vi "unweightedStats.vi"(7 "U":dbl[](array[numeric]), 9 "Data Shift Input":dbl[](array[numeric])) -> (0 "Skew":dbl, 1 "Kurt":dbl, 2 "u'/U":dbl, 3 "u^4":dbl, 4 "U":dbl, 5 "u^3":dbl, 6 "u^2":dbl, 8 "Data Shift Output":dbl[](array[numeric]))   [LabVIEW 2013]
uses:
  Globals/measurementGlobal.vi
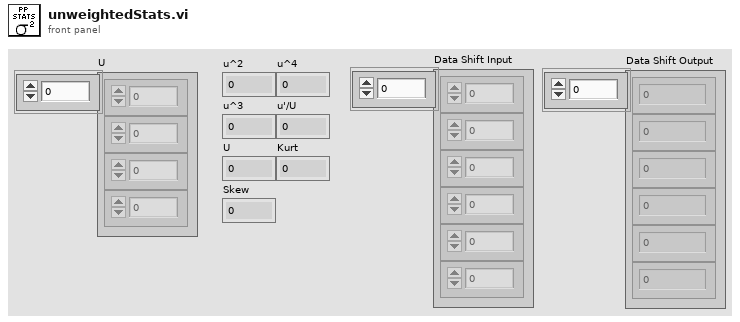
[diagram p1: front panel]
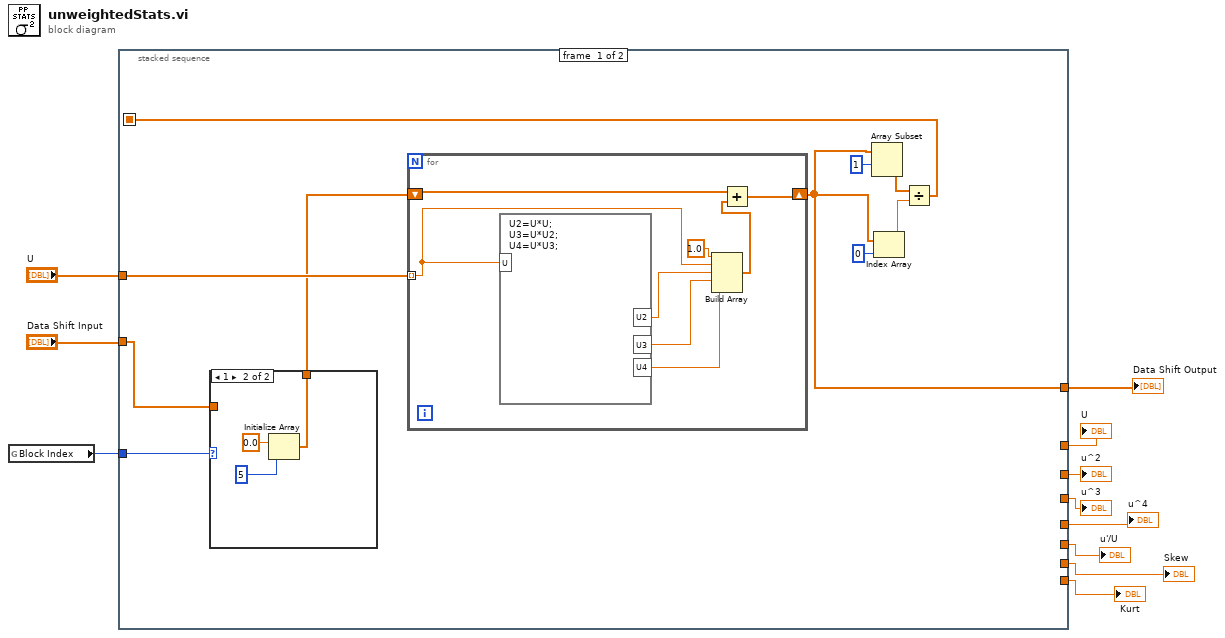
[diagram p0: block diagram]
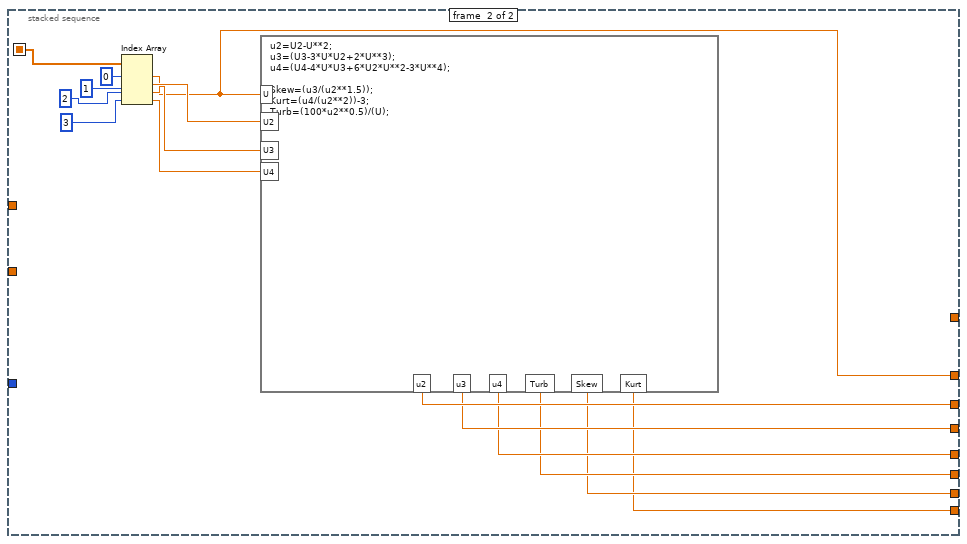
[diagram p3: hidden frame]
diagram:
  n1 = global read "measurementGlobal.vi" "Block Index"() -> (w3:i32)
  n2 = stacked-sequence {
    seq-local: [w12 _] -> [_ w48]
    tunnel: "U" -> [w21 _]
    tunnel: w3 -> [w20 _]
    tunnel: "Data Shift Input" -> [w18 _]
    tunnel: [_ w40] -> w10
    tunnel: [_ w39] -> w9
    tunnel: [_ w38] -> w8
    tunnel: [_ w37] -> w7
    tunnel: [_ w36] -> w5
    tunnel: [_ w35] -> w4
    tunnel: [_ w34] -> w6
    tunnel: [w16 _] -> w1
    frame #0 {
      n3 = case shown="1" w20 {
        tunnel: [w22 w23] -> w19
        tunnel: w18 -> [w22 _]
        frame 0, Default {
        }
        frame 1 {
          n4 = Initialize Array(0.0 ("element"), 5 ("dimension size")) -> (w23:dbl[])
        }
      }
      n5 = for {
        tunnel: w21 -> [w33] mode=indexing
        shift-right: [w27] -> w16
        shift-left: w19 -> [w28]
        n6 = formula code="U2=U*U;\nU3=U*U2;\nU4=U*U3;"("U"=w33) -> ("U2"=w32:dbl, "U3"=w31:dbl, "U4"=w30:dbl)
        n7 = Build Array(1.0 ("element"), w33, w32, w31, w30) -> (w29:dbl[])
        n8 = Add(x=w28, y=w29) -> (x+y=w27:dbl[])
      }
      n9 = Array Subset(array=w16, index=1) -> (w14:dbl[])  [unwired: 1 in]
      n10 = Index Array(array=w16, index=0) -> (element=w13:dbl)
      n11 = Divide(x=w14, y=w13) -> (x/y=w12:dbl[])
    }
    frame #1 {
      n12 = Index Array(array=w48, index #1=0 ("index"), index #2=1 ("index"), index #3=2 ("index"), index #4=3 ("index")) -> (element #1=w34:dbl, element #2=w43:dbl, element #3=w42:dbl, element #4=w41:dbl)
      n13 = formula code="u2=U2-U**2;\nu3=(U3-3*U*U2+2*U**3);\nu4=(U4-4*U*U3+6*U2*U**2-3*U**4);\n\nSkew=(u3/(u2**1.5));\nKurt=(u4/(u2**2))-3;\nTurb=(100*u2**0.5)/(U);"("U"=w34, "U2"=w43, "U3"=w42, "U4"=w41) -> ("u2"=w40:dbl, "u3"=w39:dbl, "u4"=w38:dbl, "Turb"=w37:dbl, "Skew"=w36:dbl, "Kurt"=w35:dbl)
    }
  }
  "u^2" <- w10
  "u^3" <- w9
  "u^4" <- w8
  "u'/U" <- w7
  "U" <- w6
  "Skew" <- w5
  "Kurt" <- w4
  "Data Shift Output" <- w1
